vi "test_DCPowerInstrument_InitializeSessionsWithUnregisteredSessionsReserved_RemoteSessionsInitialized.vi"(8 "error in":errorcluster) -> (0 "error out":errorcluster, 2 "result":string, 3 "pass":bool)   [LabVIEW 2020, in "MeasurementServerTests.lvlib"]
uses:
  MeasurementServerTests.lvlib
  78c0f8c1-8fe2-4936-9d85-28ac64cefb56.vi
  Runtime/MeasurementLink niDCPower/Initialize Sessions - NSess.vi
  Runtime/MeasurementLink niDCPower/MeasurementLink niDCPower.lvlib
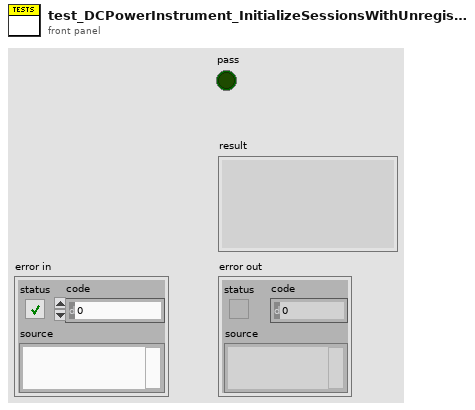
[diagram p1: front panel]
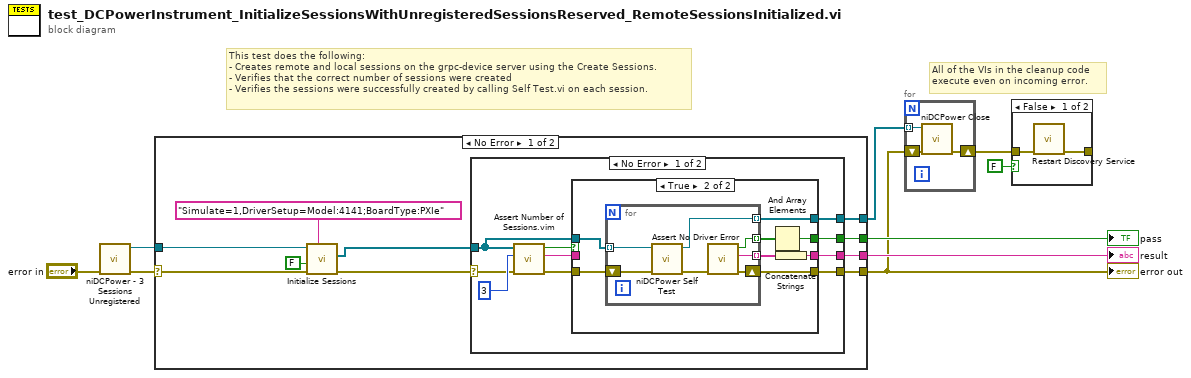
[diagram p0: block diagram]
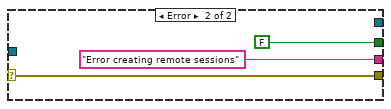
[diagram p3: hidden frame]
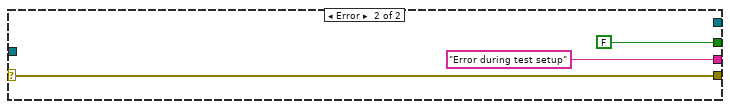
[diagram p4: hidden frame]
diagram:
  # "All of the VIs in the cleanup code\nexecute even on incoming error."
  # "This test does the following:\n- Creates remote and local sessions on the grpc-device server using the Create Sessions.\n- Verifies that the correct number of sessions were created\n- Verifies the sessions were successfully created by calling Self Test.vi on each session."
  n1 = call "niDCPower - 3 Sessions Unregistered.vi"("error in"="error in") -> ("error out"=w3:errorcluster, "session reservation out"=w2:refnum<class "Session Reservation.lvclass">)  [unwired: 9 in]
  n2 = case shown="No Error" w3 {
    selector: w3 -> [w14 w52]
    tunnel: [w18 w52] -> w5
    tunnel: [w19 FALSE] -> w6
    tunnel: [w17 "Error during test setup" ("f")] -> w9
    tunnel: [w16 _] -> w8
    tunnel: w2 -> [w15 _]
    frame No Error {
      n3 = call-poly "Initialize Sessions.vi"("option string"="Simulate=1,DriverSetup=Model:4141;BoardType:PXIe", "error in"=w14, "reset"=FALSE, "session reservation in"=w15) -> ("error out"=w11:errorcluster, "sessions"=w10:refnum<k15>[])  [unwired: 4 in, 2 out]
      n4 = case shown="No Error" w11 {
        selector: w11 -> [w23 w50]
        tunnel: [w24 FALSE] -> w19
        tunnel: [w28 w50] -> w18
        tunnel: [w29 "Error creating remote sessions"] -> w17
        tunnel: [w27 _] -> w16
        tunnel: w10 -> [w26 _]
        frame No Error {
          n5 = call "Assert Number of Sessions.vim"("error in"=w23, "expected number of sessions"=3 ("y"), "sessions"=w26) -> ("error out"=w22:errorcluster, "result"=w20:string, "pass"=w21:bool)  [unwired: 6 in]
          n6 = case shown="True" w21 {
            selector: w21 -> [w33 _]
            tunnel: [w32 w34] -> w29
            tunnel: [w31 w39] -> w28
            tunnel: [w30 w38] -> w27
            tunnel: w26 -> [w30 w37]
            tunnel: [w33 w35] -> w24
            tunnel: w22 -> [w31 w36]
            tunnel: w20 -> [w32 _]
            frame False {
            }
            frame True {
              n7 = for {
                tunnel: [w48] -> w41 mode=indexing
                tunnel: [w47] -> w40 mode=indexing
                tunnel: [w45] -> w38 mode=indexing
                tunnel: w37 -> [w43] mode=indexing
                shift-right: [w46] -> w39
                shift-left: w36 -> [w42]
                n8 = call <instrlib>:"niDCPower Self Test.vi"("error in (no error)"=w42, "instrument handle"=w43) -> ("error out"=w44:errorcluster, "instrument handle out"=w45:refnum<k15>)  [unwired: 6 in, 2 out]
                n9 = call "Assert No Driver Error.vi"("error in"=w44) -> ("error out"=w46:errorcluster, "result"=w47:string, "pass?"=w48:bool)  [unwired: 8 in]
              }
              n10 = And Array Elements(Boolean array=w41) -> (logical AND=w35:bool)
              n11 = Concatenate Strings(w40) -> (w34:string)
            }
          }
        }
        frame Error {
        }
      }
    }
    frame Error {
    }
  }
  "error out" <- w5
  "pass" <- w6
  "result" <- w9
  n12 = for {
    tunnel: w8 -> [w57] mode=indexing
    shift-right: [w56] -> w7
    shift-left: w5 -> [w55]
    n13 = call <instrlib>:"niDCPower Close.vi"("error in (no error)"=w55, "instrument handle"=w57) -> ("error out"=w56:errorcluster)  [unwired: 9 in]
  }
  n14 = case shown="False" FALSE {
    tunnel: w7 -> [w59 _]
    tunnel: [w58 _] -> _
    frame False {
      n15 = call "Restart Discovery Service.vi"("error in"=w59) -> ("error out"=w58:errorcluster)  [unwired: 10 in]
    }
    frame True {
    }
  }
